vi "test7.vi"() -> ()   [LabVIEW 2020]
uses:
  <vilib>/Platform/TimedLoop/XDataNode/timing_clust.ctl
  <vilib>/Platform/TimedLoop/XDataNode/nitl_modes.ctl
  <vilib>/Platform/TimedLoop/XDataNode/wakeup.ctl
  37583fcc-cec8-480d-a6d0-1da09da3d0dd.vi
  <vilib>/platform/TimedLoop/XDataNode/XDataNode.xnode
  <vilib>/Platform/TimedLoop/XDataNode/XDNodeRunTimeDep.lvlib
panel:
  out "Distance 2":dbl
  out "Move Time 2":u32
  in  "Array":cluster{"x":dbl, "y":dbl}[](array[cluster])
  out "Tank":dbl(slide) scale=0.0..1.0
  out "Current XY":cluster{"X":dbl, "Y":dbl}
  out "XY Graph":cluster{dbl[], dbl[]}[](graph)
  out "Stopped":bool
  in  "Stop":bool
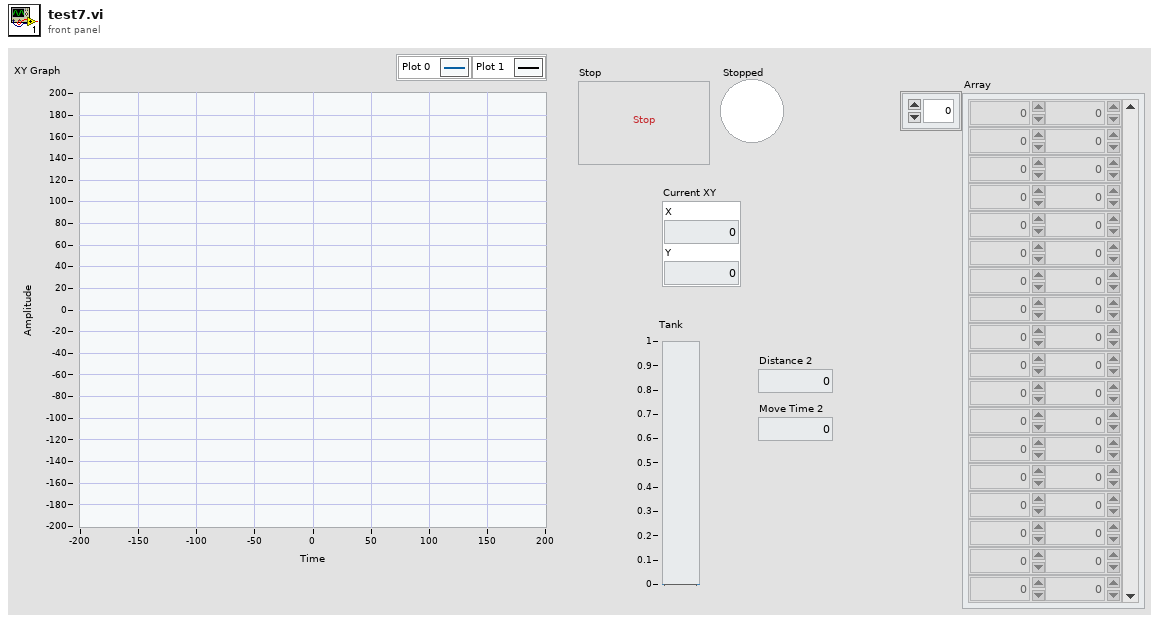
[diagram p1: front panel]
types:
  T1 = typedef "XDNodeRunTimeDep.lvlib/timing_clust.ctl" = cluster{"Expected End [f-1]":u64, "Actual End [f-1]":u64, "Finished Late? [f-1]":bool, "Expected End [i-1]":u64, "Actual End [i-1]":u64, "Finished Late? [i-1]":bool, "Expected Start [i]":u64, "Actual Start [i]":u64, "Expected Start [f]":u64, "Actual Start [f]":u64, "Source Name":string, "Structure Name":string, "Period":i64, "Deadline":i64, "Offset":i64, "Start":i64, "Priority":i32, "Timeout":i32, "Mode":T2, "Wakeup Reason":T3, "Error":errorcluster, "Source Type":string, "Secondary Source Type":string, "Global End Time":u64, "Global Start Time":u64, "Frame Duration":u64, "Iteration Duration":u64, "Assigned CPU":i32, "I/O Scan Engine Mode":u32}
  T2 = typedef "XDNodeRunTimeDep.lvlib/nitl_modes.ctl" = enum32{"No Change", "Process missed periods, maintain original phase", "Discard missed periods, maintain original phase", "Process missed periods, ignore original phase", "Discard missed periods, ignore original phase"}
  T3 = typedef "XDNodeRunTimeDep.lvlib/wakeup.ctl" = enum32{"Normal", "Aborted", "Asynchronous wakeup", "Timing source error", "Timed loop error", "Timeout"}
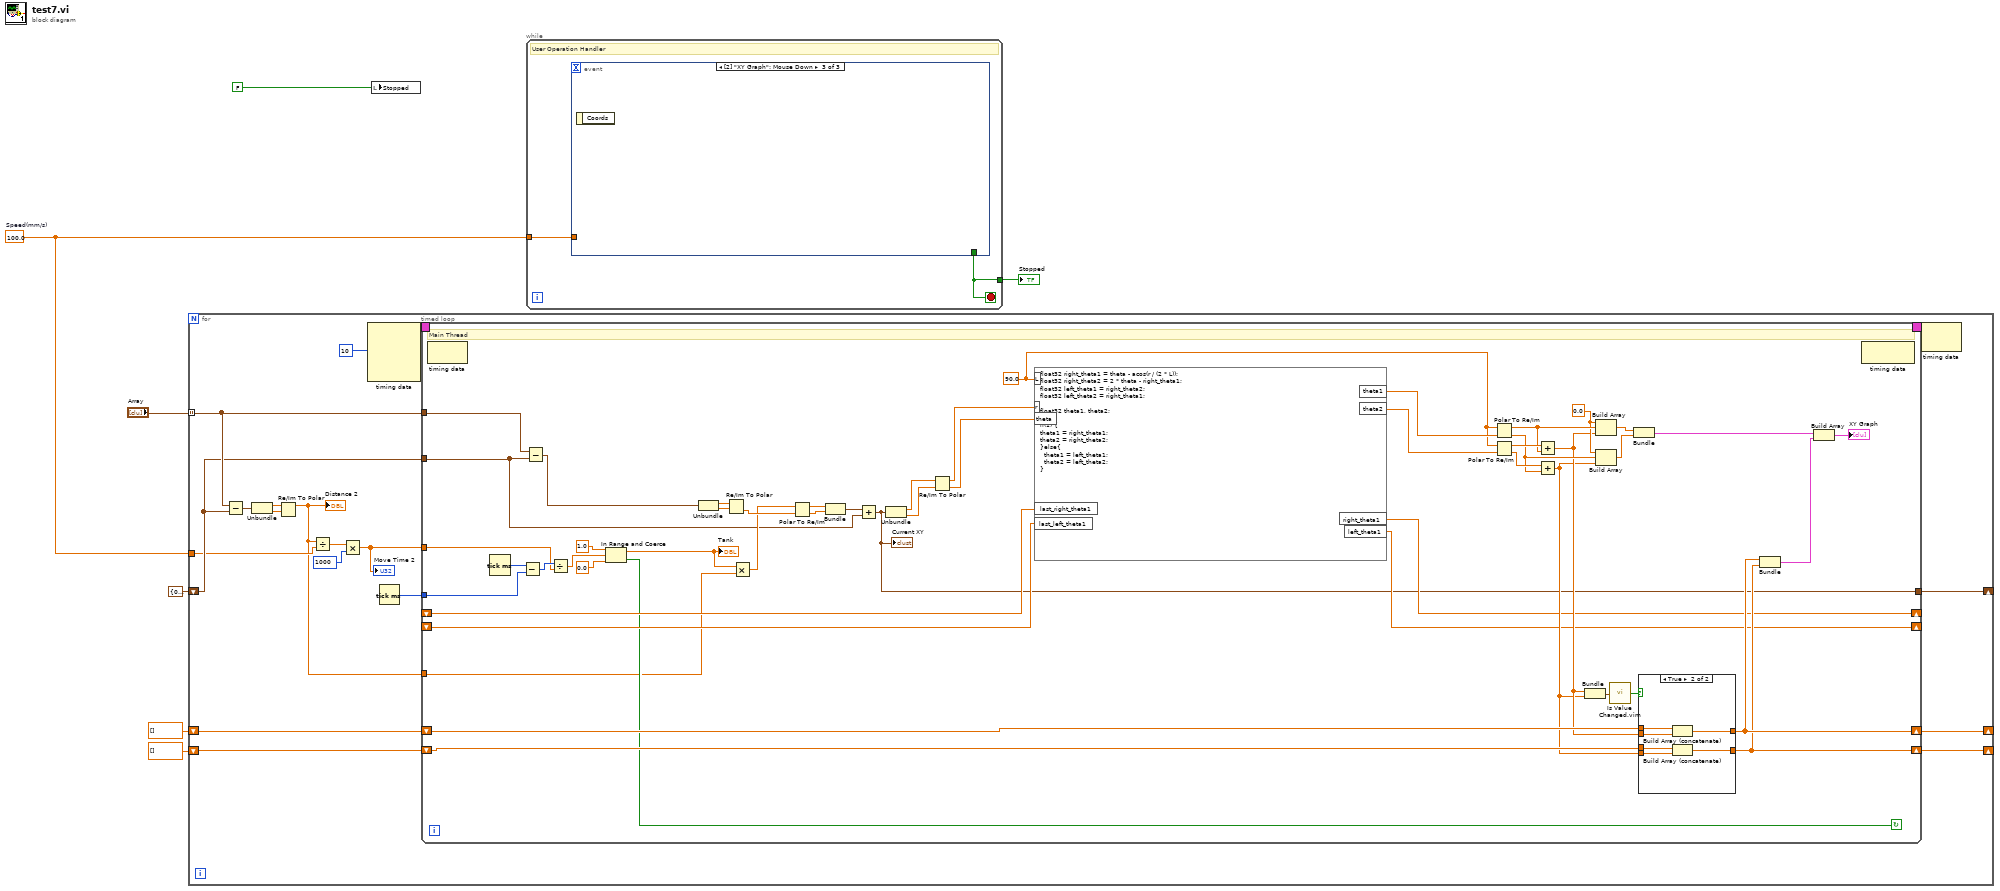
[diagram p0: block diagram]
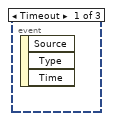
[diagram p3: hidden frame]
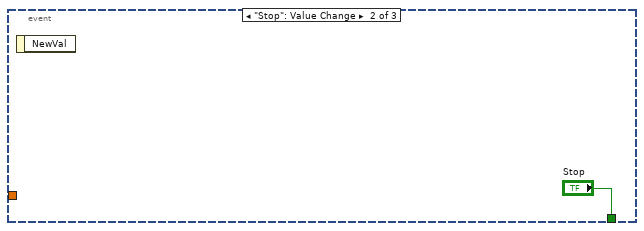
[diagram p4: hidden frame]
diagram:
  w3 = 100.0  # Speed(mm/s)
  n1 = for {
    tunnel: "Array" -> [w17] mode=indexing
    shift-right: [w23] -> _
    shift-left: cluster{dbl, dbl} {0.0, 0.0} -> [w16]
    tunnel: w3 -> [w15]
    shift-right: [w10] -> _
    shift-left: dbl[] [] -> [w11]
    shift-right: [w9] -> _
    shift-left: dbl[] [] -> [w8]
    n2 = Subtract(x=w17, y=w16) -> (x-y=w20:cluster{dbl, dbl})
    n3 = Unbundle(w20) -> (w19:dbl, w18:dbl)
    n4 = Re/Im To Polar(2:w18, 3:w19) -> (1:w13:dbl)  [unwired: 1 out]
    "Distance 2" <- w13
    n5 = Divide(x=w13, y=w15) -> (x/y=w21:dbl)
    n6 = Multiply(x=w21, y=u32 1000 ("millisecond timer value")) -> (x*y=w14:dbl)
    "Move Time 2" <- w14
    n7 = node-c288(i64 10 ("Period")) -> (w26:T1)  [unwired: 3 in]
    n8 = Tick Count (ms)() -> (millisecond timer value=w12:u32)
    n9 = timed-loop {
      timing: w26 -> [_]
      timing-out: [_] -> w25
      shift-right: [w46] -> w10
      shift-left: w11 -> [w53]
      shift-right: [w45] -> w9
      shift-left: w8 -> [w52]
      shift-right: [w36] -> _
      shift-left: _ -> [w35]
      shift-right: [w37] -> _
      shift-left: _ -> [w34]
      tunnel: w17 -> [w32]
      tunnel: [w31] -> w23
      tunnel: w16 -> [w30]
      tunnel: w14 -> [w29]
      tunnel: w13 -> [w28]
      tunnel: w12 -> [w27]
      stop <- w33 continue-if-true
      w57 = 0.0 ("element")
      w54 = 90.0 ("input variable")
      # "Main Thread"
      n10 = node-c288() -> ()  [unwired: 1 in, 1 out]
      n11 = Tick Count (ms)() -> (millisecond timer value=w76:u32)
      n12 = Subtract(x=w76, y=w27) -> (x-y=w42:u32)
      n13 = Subtract(x=w32, y=w30) -> (x-y=w75:cluster{dbl, dbl})
      n14 = Divide(x=w42, y=w29) -> (x/y=w41:dbl)
      n15 = In Range and Coerce(upper limit=1.0 ("lower limit"), x=w41, lower limit=0.0) -> (coerced(x)=w38:dbl, In Range?=w33:bool)
      "Tank" <- w38
      n16 = Unbundle(w75) -> (w74:dbl, w73:dbl)
      n17 = Re/Im To Polar(2:w73, 3:w74) -> (0:w72:dbl)  [unwired: 1 out]
      n18 = Multiply(x=w38, y=w28) -> (x*y=w65:dbl)
      n19 = Polar To Re/Im(2:w72, 3:w65) -> (0:w70:dbl, 1:w71:dbl)
      n20 = Bundle(w71, w70) -> (w69:cluster{dbl, dbl})  [unwired: 1 in]
      n21 = Add(x=w69, y=w30) -> (x+y=w31:cluster{dbl, dbl})
      "Current XY" <- w31
      n22 = Unbundle(w31) -> (w68:dbl, w67:dbl)
      n23 = Re/Im To Polar(2:w67, 3:w68) -> (0:w66:dbl, 1:w64:dbl)
      n24 = formula code="float32 right_theta1 = theta - acos(r / (2 * L));\nfloat32 right_theta2 = 2 * theta - right_theta1;\nfloat32 left_theta1 = right_theta2;\nfloat32 left_theta2 = right_theta1;\n\nfloat32 theta1, theta2;\n\nif(1) {\ntheta1 = right_theta1;\ntheta2 = right_theta2;\n}else{\n  theta1 = left_theta1;\n  theta2 = left_theta2;\n}"("r"=w64, "theta"=w66, "L"=w54, "last_right_theta1"=w35, "last_left_theta1"=w34) -> ("theta1"=w56:sgl, "theta2"=w55:sgl, "right_theta1"=w36:sgl, "left_theta1"=w37:sgl)
      n25 = Polar To Re/Im(2:w56, 3:w54) -> (0:w60:dbl, 1:w61:dbl)
      n26 = Polar To Re/Im(2:w55, 3:w54) -> (0:w62:dbl, 1:w63:dbl)
      n27 = Add(x=w63, y=w61) -> (x+y=w51:dbl)
      n28 = Add(x=w62, y=w60) -> (x+y=w50:dbl)
      n29 = Bundle(w51, w50) -> (w49:cluster{dbl, dbl})  [unwired: 1 in]
      n30 = Build Array(w57, w61, w51) -> (w59:dbl[])
      n31 = Build Array(w57, w60, w50) -> (w58:dbl[])
      n32 = call "Is Value Changed.vim"("value"=w49) -> ("changed or first call?"=w48:bool)
      n33 = Bundle(w59, w58) -> (w47:cluster{dbl[], dbl[]})  [unwired: 1 in]
      n34 = case shown="True" w48 {
        tunnel: w51 -> [_ w84]
        tunnel: w50 -> [_ w83]
        tunnel: [w78 w82] -> w46
        tunnel: [w77 w81] -> w45
        tunnel: w53 -> [w78 w80]
        tunnel: w52 -> [w77 w79]
        frame False {
        }
        frame True {
          n35 = Build Array (concatenate)(w80, w84) -> (w82:dbl[])
          n36 = Build Array (concatenate)(w79, w83) -> (w81:dbl[])
        }
      }
      n37 = Bundle(w46, w45) -> (w44:cluster{dbl[], dbl[]})  [unwired: 1 in]
      n38 = Build Array(w47, w44) -> (→"XY Graph":cluster{dbl[], dbl[]}[])
      n39 = node-c288() -> ()  [unwired: 1 in, 1 out]
    }
    n40 = node-c288(w25) -> ()  [unwired: 1 out]
  }
  n41 = local write "Stopped"(FALSE ("Stopped")) -> ()
  n42 = while {
    tunnel: [w92] -> w7
    tunnel: w3 -> [w91]
    stop <- w92 stop-if-true
    # "User Operation Handler"
    n43 = event shown="[2] \"XY Graph\": Mouse Down" {
      selector: _ -> [_ _ _]
      dyn-events: _ -> [_ _ _]
      timeout: _ -> [_ _ _]
      tunnel: [_ "Stop" _] -> w92
      tunnel: w91 -> [_ _ _]
      event Timeout {
        n44 = event-data() -> ()  [unwired: 1 in, 3 out]
      }
      event "Stop": Value Change {
        n45 = event-data() -> ()  [unwired: 1 in, 1 out]
      }
      event "XY Graph": Mouse Down {
        n46 = event-data() -> ()  [unwired: 1 in, 1 out]
      }
    }
  }
  "Stopped" <- w7
